vi "That was easy!.vi"(8 "error in (no error)":errorcluster, 11 "FPGA VI Reference in":T1) -> (0 "error out":errorcluster, 3 "FPGA VI Reference out":T1)   [LabVIEW 2009]
uses:
  TypeDefs/Sensor TypeDefs/FPGA Main ref.ctl
  <vilib>/rvi/interface/nirviMethod/nirviMethod.xnode
  FPGA Bitfiles/Q_IGVC_2010.lvproj_FPGA Target_FPGA_MAIN.vi.lvbitx
  <vilib>/LabVIEW Targets/FPGA/RIO/nirio_HostInterface/nirio_WaitOnIRQ.vi
  <vilib>/RVI Host/nirviSupport.llb/nirviErrorClusterFromErrorCode.vi
  <vilib>/rvi/interface/common/niFpgaNodeNameForErrorReporting.ctl
  <vilib>/rvi/errors/niLvFpgaWhatHappensToTopLevelVI.ctl
  <vilib>/rvi/errors/niLvFpgaAdjustHostInterfaceError.vi
  <vilib>/Utility/error.llb/Error Cluster From Error Code.vi
  <vilib>/rvi/interface/nirviReadWriteControl/nirviReadWriteControl.xnode
  NiRioSrv.dll
panel:
  out "IRQ(s) Asserted":i32
  out "Timed Out":bool
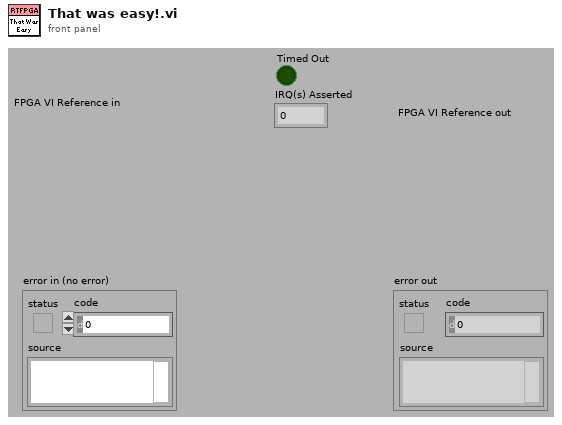
[diagram p1: front panel]
types:
  T1 = typedef "FPGA Main ref.ctl" = refnum<k20>
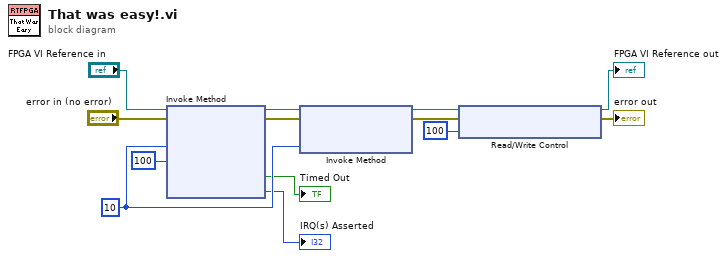
[diagram p0: block diagram]
diagram:
  w9 = 10 ("IRQ Number(s)")
  n1 = xnode "Invoke Method"("FPGA VI Reference In"="FPGA VI Reference in", "error in"="error in (no error)", "IRQ Number(s)"=w9, "Timeout (ms)"=100) -> ("FPGA VI Reference Out"=w12:T1, "error out"=w11:errorcluster, "Timed Out"=→"Timed Out":bool, "IRQ(s) Asserted"=→"IRQ(s) Asserted":i32)
  n2 = xnode "Invoke Method"("FPGA VI Reference In"=w12, "error in"=w11, "IRQ Number(s)"=w9) -> ("FPGA VI Reference Out"=w3:T1, "error out"=w6:errorcluster)
  n3 = xnode "Read/Write Control"("FPGA VI Reference In"=w3, "error in"=w6, "That Was Easy Duration"=u32 100) -> ("FPGA VI Reference Out"=→"FPGA VI Reference out":T1, "error out"=→"error out":errorcluster)
